vi "ball status fg.vi"(1 "Menu":T1, 2 "Ball State":enum16{"no ball", "holding", "loaded"}(ring)) -> (0 "Ball State":enum16{"no ball", "holding", "loaded"}(ring))   [LabVIEW 2013]
uses:
  typedefs/fg_typedef.ctl
panel:
  # "An Average Functional Global with Some Ball Status Information"
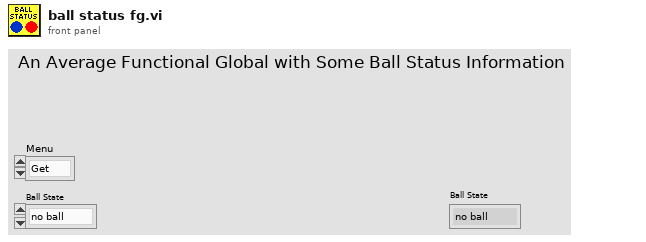
[diagram p1: front panel]
types:
  T1 = typedef "fg_typedef.ctl" = enum16{"Get", "Set"}
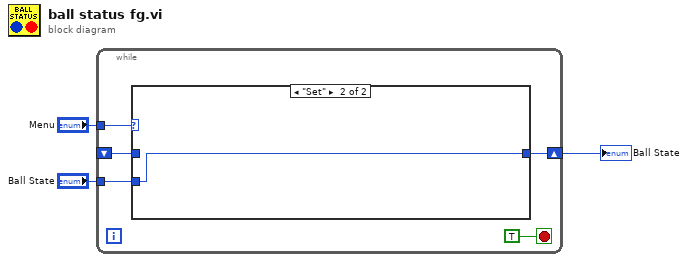
[diagram p0: block diagram]
diagram:
  n1 = while {
    tunnel: "Menu" -> [w8]
    tunnel: "Ball State" -> [w7]
    shift-right: [w6] -> w1
    shift-left: _ -> [w5]
    stop <- TRUE stop-if-true
    n2 = case shown="\"Set\"" w8 {
      tunnel: w7 -> [_ w10]
      tunnel: [w9 w10] -> w6
      tunnel: w5 -> [w9 _]
      frame "Get", Default {
      }
      frame "Set" {
      }
    }
  }
  "Ball State" <- w1
